vi "uTransport_uActor_Get_Queue.vi"(11 "uTransport_uActor in":refnum<class "uTransport_uActor.lvclass">) -> (2 "Actor Queue":refnum<queue>)   [LabVIEW 2023, in "uLib.lvlib" / "uTransport_uActor.lvclass"]
uses:
  uTransport_uActor.lvclass
  uMsg/uMsg/uMsg.lvclass
  uTransport_uActor.lvclass/uTransport_uActor.ctl
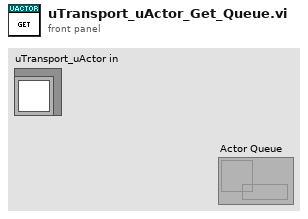
[diagram p1: front panel]
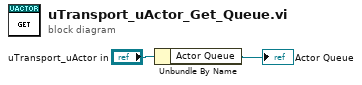
[diagram p0: block diagram]
diagram:
  n1 = Unbundle By Name("uTransport_uActor in") -> ("Actor Queue"=→"Actor Queue":refnum<queue>)
